vi "Upload Photo.vi"(6 "Photo tags":string, 7 "Album Cover":string, 8 "Description":string="just testing", 9 "Photoset Name":string="Photobooth Testing", 10 "Image Path":string, 11 "Flickr Ref":refnum<k24>) -> (3 "Flickr Ref out":refnum<k24>)   [LabVIEW 2012]
uses:
  C:/Users/telsey/Desktop/Personal Projects/Photobooth/Flickr API/FlickrNet-3.5.0/FlickrNet.dll
  FlickrNet-3.5.0/FlickrNet.dll
panel:
  out "error out":errorcluster
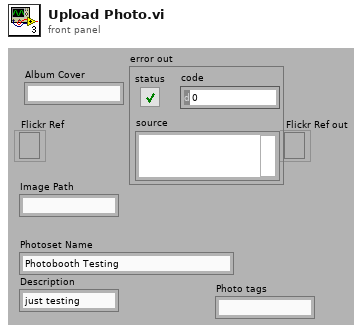
[diagram p1: front panel]
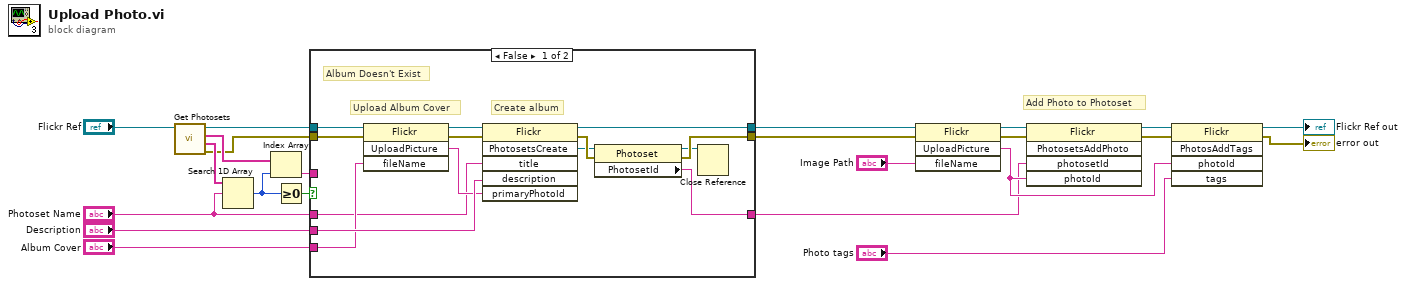
[diagram p0: block diagram]
diagram:
  # "Add Photo to Photoset"
  n1 = call "Get Photosets.vi"("Flickr Ref"="Flickr Ref") -> ("error out"=w8:errorcluster, "Names"=w17:string[], "ids"=w16:string[], "Flickr Ref out"=w18:refnum<k24>)  [unwired: 7 in]
  n2 = Search 1D Array(1D array=w17, element="Photoset Name") -> (index of element=w21:i32)  [unwired: 1 in]
  n3 = Index Array(array=w16, index=w21) -> (element=w22:string)
  n4 = Greater Or Equal To 0?(x=w21) -> (x >= 0?=w20:bool)
  n5 = case shown="False" w20 {
    tunnel: w18 -> [w36 w40]
    tunnel: w22 -> [_ w38]
    tunnel: [w29 w40] -> w2
    tunnel: "Photoset Name" -> [w27 _]
    tunnel: "Description" -> [w37 _]
    tunnel: "Album Cover" -> [w33 _]
    tunnel: [w26 w38] -> w3
    tunnel: w8 -> [w32 w39]
    tunnel: [w28 w39] -> w1
    frame False {
      # "Album Doesn't Exist"
      # "Upload Album Cover"
      # "Create album"
      n6 = invoke class="Flickr" method="UploadPicture"(reference=w36, error in=w32, "fileName"=w33) -> (reference out=w35:refnum<k24>, error out=w31:errorcluster, "UploadPicture"=w34:string)  [unwired: 1 in, 1 out]
      n7 = invoke class="Flickr" method="PhotosetsCreate"(reference=w35, error in=w31, "title"=w27, "description"=w37, "primaryPhotoId"=w34) -> (reference out=w29:refnum<k24>, error out=w30:errorcluster, "PhotosetsCreate"=w25:refnum<k24>)  [unwired: 1 in, 3 out]
      n8 = property class="Photoset"(reference=w25, error in=w30) -> (reference out=w24:refnum<k24>, error out=w28:errorcluster, "PhotosetId"=w26:string)
      n9 = Close Reference(reference=w24) -> ()  [unwired: 1 in, 1 out]
    }
    frame True {
    }
  }
  n10 = invoke class="Flickr" method="UploadPicture"(reference=w2, error in=w1, "fileName"="Image Path") -> (reference out=w6:refnum<k24>, error out=w7:errorcluster, "UploadPicture"=w12:string)  [unwired: 1 in, 1 out]
  n11 = invoke class="Flickr" method="PhotosetsAddPhoto"(reference=w6, error in=w7, "photosetId"=w3, "photoId"=w12) -> (reference out=w10:refnum<k24>, error out=w5:errorcluster)  [unwired: 1 in, 3 out]
  n12 = invoke class="Flickr" method="PhotosAddTags"(reference=w10, error in=w5, "photoId"=w12, "tags"="Photo tags") -> (reference out=→"Flickr Ref out":refnum<k24>, error out=→"error out":errorcluster)  [unwired: 1 in, 3 out]
